vi "3_5_3.vi"() -> ()   [LabVIEW 2012]
panel:
  out "Array 3":i32[][](array[numeric])
  in  "Numeric":i32
  in  "Array 2":i32[][](array[numeric])
  in  "stop":bool
  in  "OK Button":bool
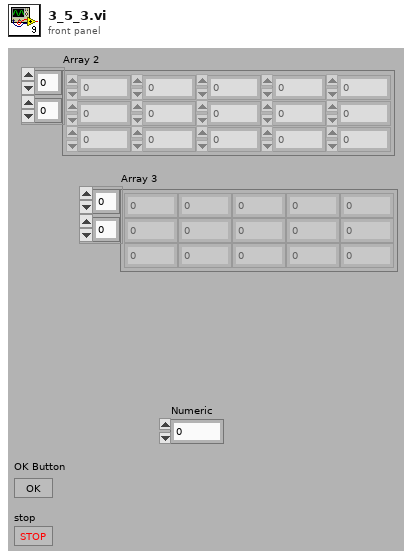
[diagram p1: front panel]
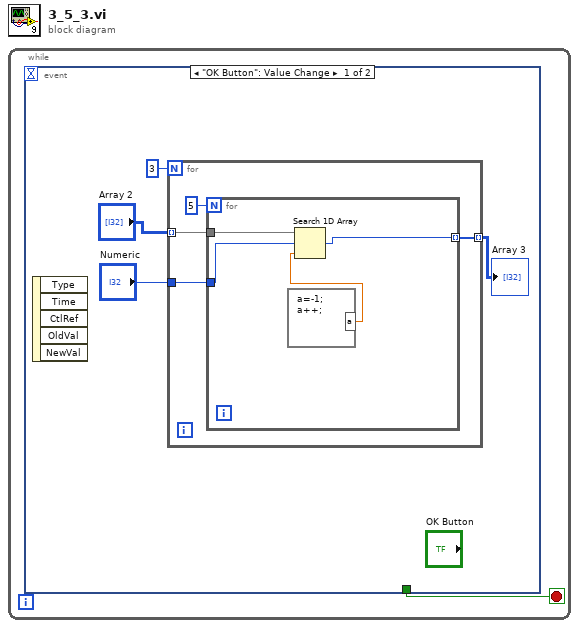
[diagram p0: block diagram]
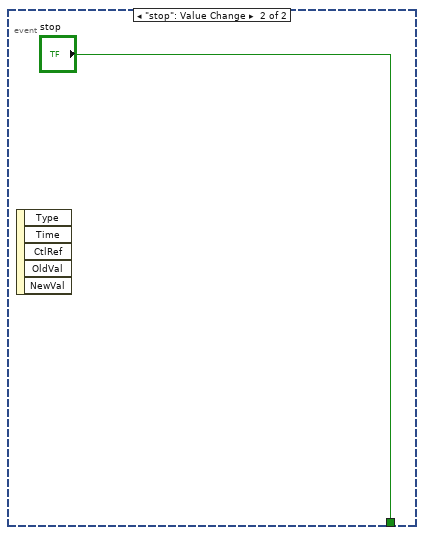
[diagram p2: hidden frame]
diagram:
  n1 = while {
    stop <- w1 stop-if-true
    n2 = event shown="[0] \"OK Button\": Value Change" {
      selector: _ -> [_ _]
      dyn-events: _ -> [_ _]
      timeout: _ -> [_ _]
      tunnel: [_ "stop"] -> w1
      event "OK Button": Value Change {
        n3 = event-data() -> ()  [unwired: 1 in, 5 out]
        n4 = for {
          N: 3 -> [_]
          tunnel: "Array 2" -> [w9] mode=indexing
          tunnel: "Numeric" -> [w8]
          tunnel: [w7] -> w2 mode=indexing
          n5 = for {
            N: 5 -> [_]
            tunnel: w9 -> [w13]
            tunnel: w8 -> [w12]
            tunnel: [w11] -> w7 mode=indexing
            n6 = formula code="a=-1;\na++;"() -> ("a"=w10:dbl)
            n7 = Search 1D Array(1D array=w13, element=w12, start index (0)=w10) -> (index of element=w11:i32)
          }
        }
        "Array 3" <- w2
      }
      event "stop": Value Change {
        n8 = event-data() -> ()  [unwired: 1 in, 5 out]
      }
    }
  }
